vi "CIMAQ Overlay ROI Big.vi"(6 "Overlay Thickness":i32(slide)=5 scale=0.0..20.0, 7 "Color":u32(colorbox)=16711680, 8 "error in (no error)":errorcluster, 9 "Max number of vectors in ROI":i32=9999, 10 "ROI Descriptor":T1 {"Contours"."Type" items=["No Selection", "Point", "Line", "Rectangle", "Oval", "Polygon", "Freehand Region", "Annulus", "Unused2", "Unused3", "Broken Line", "Freehand Line", "Rotated Rectangle"]}, 11 "Image In":T2) -> (0 "error out":errorcluster, 3 "Image Out":T2)   [LabVIEW 2014]
uses:
  <vilib>/vision/Image Controls.llb/IMAQ Image.ctl
  <vilib>/vision/NI_Vision_Development_Module.lvlib
panel:
  in  "OverlayName":string
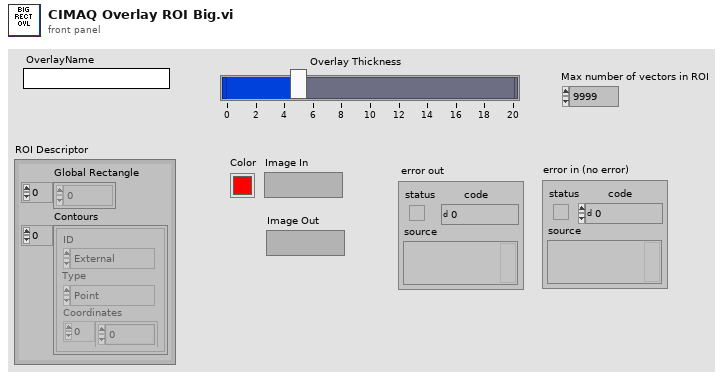
[diagram p1: front panel]
types:
  T1 = typedef "ROI Descriptor" = cluster{"Global Rectangle":i32[], "Contours":cluster{"ID":enum32{"External", "Internal"}, "Type":u32, "Coordinates":i32[]}[]}
  T2 = typedef "IMAQ Image.ctl" = refnum<image>
  T3 = enum32{"AutoM", "Close", "Dilate", "Erode", "Gradient", "Gradient out", "Gradient in", "Hit miss", "Open", "PClose", "POpen", "Thick", "Thin"}
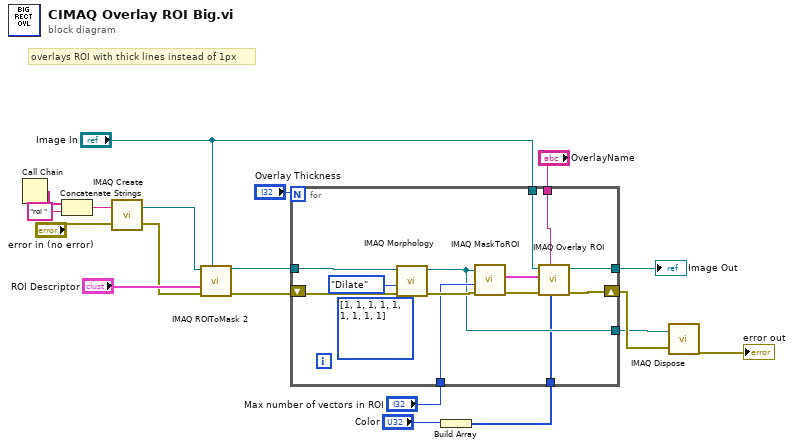
[diagram p0: block diagram]
diagram:
  # "overlays ROI with thick lines instead of 1px"
  n1 = Call Chain() -> (call chain=w17:string[])
  n2 = Concatenate Strings(w17, "roi " ("string")) -> (w16:string)
  n3 = call "IMAQ Create"("Image Name"=w16, "error in (no error)"="error in (no error)") -> ("New Image"=w6:T2, "error out"=w14:errorcluster)  [unwired: 3 in]
  n4 = call "IMAQ ROIToMask 2"("Image Model"="Image In", "error in (no error)"=w14, "ROI Descriptor"="ROI Descriptor", "Image"=w6) -> ("error out"=w11:errorcluster, "Image Out"=w13:T2)  [unwired: 5 in, 1 out]
  n5 = Build Array("Color") -> (w2:u32[])
  n6 = for {
    N: "Overlay Thickness" -> [_]
    tunnel: w13 -> [w33]
    tunnel: "Max number of vectors in ROI" -> [w27]
    shift-right: [w26] -> w7
    shift-left: w11 -> [w28]
    tunnel: [w25] -> w9
    tunnel: "Image In" -> [w24]
    tunnel: [w23] -> w5
    tunnel: w2 -> [w22]
    tunnel: "OverlayName" -> [w20]
    n7 = call "IMAQ Morphology"("Structuring Element"=i32[][] [[1, 1, 1], [1, 1, 1], [1, 1, 1]], "error in (no error)"=w28, "Operation"=T3."Dilate", "Image Src"=w33) -> ("error out"=w29:errorcluster, "Image Dst Out"=w23:T2)  [unwired: 6 in]
    n8 = call "IMAQ MaskToROI"("Image"=w23, "Max number of vectors in ROI"=w27, "error in (no error)"=w29) -> ("ROI Descriptor"=w30:T1, "error out"=w31:errorcluster)  [unwired: 4 in, 1 out]
    n9 = call "IMAQ Overlay ROI"("Colors (Green)"=w22, "Group"=w20, "error in (no error)"=w31, "ROI Descriptor"=w30, "Image"=w24) -> ("error out"=w26:errorcluster, "Image Out"=w25:T2)  [unwired: 5 in]
  }
  "Image Out" <- w9
  n10 = call "IMAQ Dispose"("Image"=w5, "error in (no error)"=w7) -> ("error out"=→"error out":errorcluster)  [unwired: 4 in]
